vi "CameraSettingsMenu.vi"() -> ()   [LabVIEW 2019]
uses:
  CameraSettings.ctl
  GlobalCamSettings.vi
  GlobalCamSettingsExperiment.vi
  Global.lvlib
panel:
  in  "Tab Control":enum32{"Continuous", "Experiment"}(tab)
  in  "Camera Settings":T1={"EM Gain :"=100.0, "Pre Amp Gain :"=1.0, "VS Speed [Index] :"=1.0, "VS Amplitude :"=1.0, "Exposure Time [s] :"=0.2, "Temperature :"=0.0, "HS Speed [s]"=1.0, "Gain > 300 :"=FALSE}
  in  "Camera Settings Exp":T1={"EM Gain :"=100.0, "Pre Amp Gain :"=1.0, "VS Speed [Index] :"=1.0, "VS Amplitude :"=1.0, "Exposure Time [s] :"=0.3, "Temperature :"=0.0, "HS Speed [s]"=1.0, "Gain > 300 :"=FALSE}
  in  "Close":bool
  in  "Help":bool
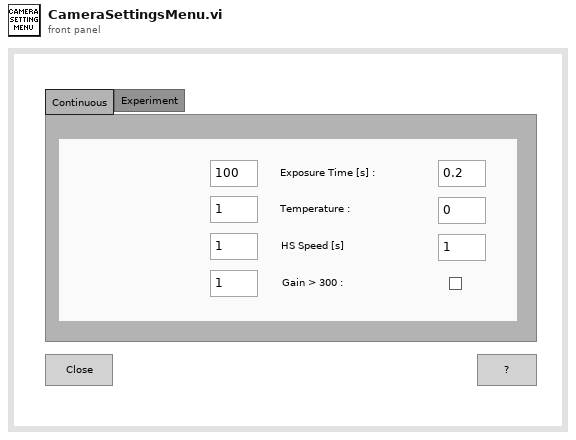
[diagram p1: front panel]
types:
  T1 = typedef "CameraSettings.ctl" = cluster{"EM Gain :":dbl, "Pre Amp Gain :":dbl, "VS Speed [Index] :":dbl, "VS Amplitude :":dbl, "Exposure Time [s] :":dbl, "Temperature :":dbl, "HS Speed [s]":dbl, "Gain > 300 :":bool}
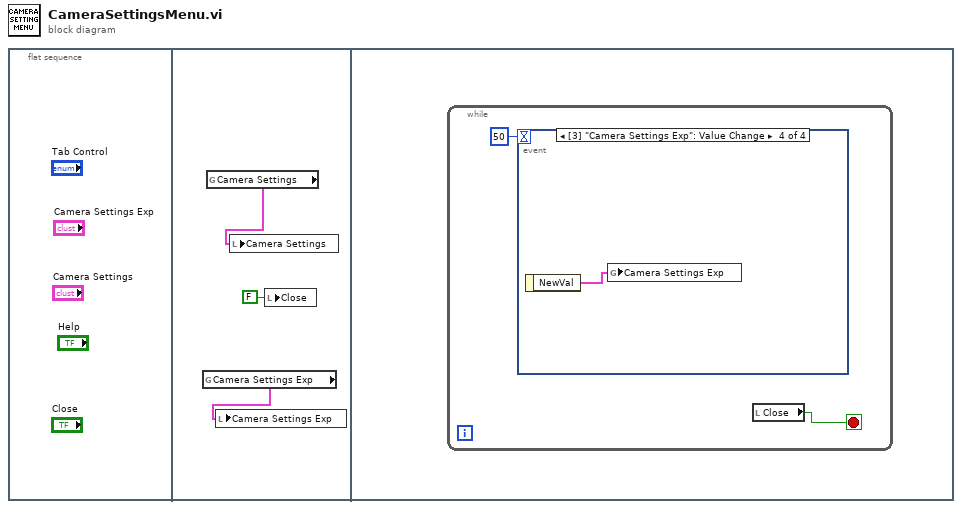
[diagram p0: block diagram]
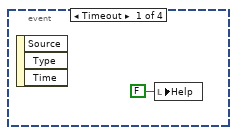
[diagram p2: hidden frame]
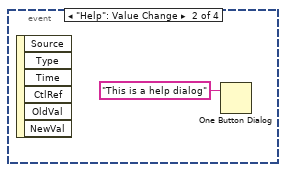
[diagram p3: hidden frame]
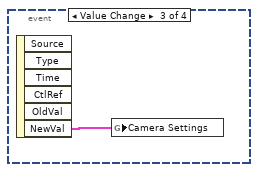
[diagram p4: hidden frame]
diagram:
  n1 = flat-sequence {
    frame #0 {
    }
    frame #1 {
      n2 = global read "GlobalCamSettingsExperiment.vi" "Camera Settings Exp"() -> (w1:T1)
      n3 = global read "GlobalCamSettings.vi" "Camera Settings"() -> (w2:T1)
      n4 = local write "Camera Settings Exp"(w1) -> ()
      n5 = local write "Camera Settings"(w2) -> ()
      n6 = local write "Close"(FALSE ("Help")) -> ()
    }
    frame #2 {
      n7 = while {
        stop <- w4 stop-if-true
        n8 = event shown="[3] \"Camera Settings Exp\": Value Change" {
          selector: _ -> [_ _ _ _]
          dyn-events: _ -> [_ _ _ _]
          timeout: 50 -> [_ _ _ _]
          event Timeout {
            n9 = event-data() -> ()  [unwired: 1 in, 3 out]
            n10 = local write "Help"(FALSE ("Help")) -> ()
          }
          event "Help": Value Change {
            n11 = event-data() -> ()  [unwired: 1 in, 6 out]
            n12 = One Button Dialog(message="This is a help dialog") -> ()  [unwired: 1 in, 1 out]
          }
          event Value Change {
            n13 = event-data() -> ("NewVal"=w8:T1)  [unwired: 1 in, 5 out]
            n14 = global write "GlobalCamSettings.vi" "Camera Settings"(w8) -> ()
          }
          event Value Change {
            n15 = event-data() -> ("NewVal"=w9:T1)  [unwired: 1 in]
            n16 = global write "GlobalCamSettingsExperiment.vi" "Camera Settings Exp"(w9) -> ()
          }
        }
        n17 = local read "Close"() -> (w4:bool)
      }
    }
  }
